vi "test Add Get and Remove Timestamp Channel.vi"(8 "error in":errorcluster, 11 "TestCase in":refnum<class "Scripting.lvclass">) -> (0 "error out":errorcluster, 3 "TestCase out":refnum<class "Scripting.lvclass">)   [LabVIEW 2020, in "Scripting.lvclass"]
uses:
  Scripting.lvclass
  <vilib>/NI VeriStand/Custom Device API/Custom Device Item Ref.ctl
  Shared/Direction.ctl
  Shared/SDI.ctl
  Scripting.lvclass/Scripting.ctl
  <vilib>/addons/_JKI Toolkits/VI Tester/TestCase.llb/TestCase.lvclass
  Scripting/AIM/AIM ARINC 429 Scripting.lvlib
  <vilib>/NI VeriStand/Custom Device API/Custom Device API.lvlib
  Shared/Transfer Speed.ctl
  C:/Program Files (x86)/National Instruments/LabVIEW 2020/vi.lib/addons/_JKI Toolkits/VI Tester/TestCase.llb/TestCase.lvclass
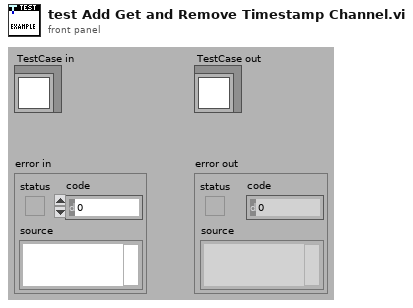
[diagram p1: front panel]
types:
  T1 = typedef "Transfer Speed.ctl" = enum16{"LO (12.5 kb/s)", "HI (100 kb/s)"}
  T2 = cluster{"SDI":bool, "SSM":bool, "Parity":bool, "Timestamp":bool}
  T3 = typedef "Direction.ctl" = enum16{"Rx", "Tx"}
  T4 = typedef "Custom Device API.lvlib/Custom Device Item Ref.ctl" = u64
  T5 = typedef "SDI.ctl" = i32
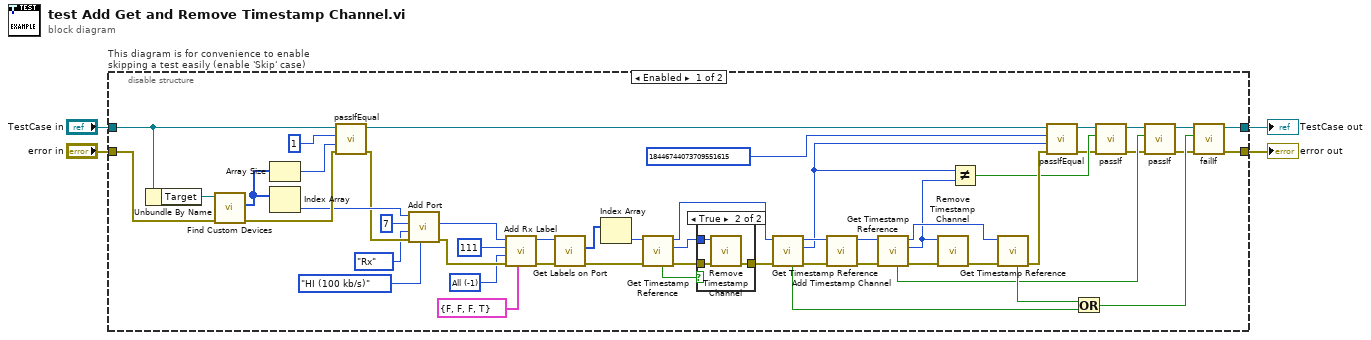
[diagram p0: block diagram]
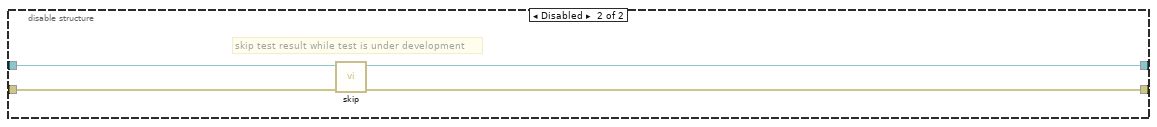
[diagram p3: hidden frame]
diagram:
  n1 = disable-structure "This diagram is for convenience to enable skipping a test easily (enable 'Skip' case)" shown="Enabled" {
    disable-tunnel: "TestCase in" -> [w55 w64]
    disable-tunnel: [w24 w62] -> w1
    disable-tunnel: [w25 w63] -> w3
    disable-tunnel: "error in" -> [w54 w61]
    frame Enabled {
      w6 = T5 -1 items=["All"=-1, "0 (b00)"=0, "1 (b01)"=1, "2 (b10)"=2, "3 (b11)"=3] ("SDI value")
      n2 = Unbundle By Name(w55) -> ("Target"=w56:refnum<k24>)
      n3 = call "Find Custom Devices.vi"("error in"=w54, "target in"=w56) -> ("error out"=w48:errorcluster, "AIM ARINC 429 custom devices"=w50:u64[])  [unwired: 7 in, 1 out]
      n4 = Array Size(array=w50) -> (size(s)=w52:i32)
      n5 = Index Array(array=w50) -> (element=w16:u64)  [unwired: 1 in]
      n6 = call-dynamic "passIfEqual.vi"("error in (no error)"=w48, "y"=w52, "x"=1 ("size(s)"), "TestCase in"=w55) -> ("error out"=w14:errorcluster, "TestCase out"=w49:refnum<class "Scripting.lvclass">)  [unwired: 6 in]
      n7 = call "Add Port.vi"("speed"=Transfer_Speed."HI (100 kb/s)", "error in"=w14, "direction"=Direction."Rx", "port number"=u16 7, "AIM ARINC 429 custom device in"=w16) -> ("error out"=w10:errorcluster, "port"=w12:T4)  [unwired: 4 in, 1 out]
      n8 = call "Add Rx Label.vi"("create channels"=T2 {"SDI"=FALSE, "SSM"=FALSE, "Parity"=FALSE, "Timestamp"=TRUE}, "error in"=w10, "SDI value"=w6, "label value"=u32 111, "port in"=w12) -> ("error out"=w9:errorcluster, "port out"=w11:T4)  [unwired: 4 in, 1 out]
      n9 = call "Get Labels on Port.vi"("error in"=w9, "port in"=w11) -> ("error out"=w31:errorcluster, "labels"=w51:T4[])  [unwired: 6 in, 2 out]
      n10 = Index Array(array=w51) -> (element=w32:T4)  [unwired: 1 in]
      n11 = call "Get Timestamp Reference.vi"("error in"=w31, "label ref in"=w32) -> ("error out"=w30:errorcluster, "timestamp channel reference"=w33:T4, "label ref out"=w29:T4, "timestamp channel found?"=w17:bool)  [unwired: 6 in]
      n12 = case shown="True" w17 {
        tunnel: w33 -> [_ w60]
        tunnel: w30 -> [w57 w59]
        tunnel: [w57 w58] -> w18
        frame False {
        }
        frame True {
          n13 = call "Remove Timestamp Channel.vi"("error in"=w59, "timestamp channel ref"=w60) -> ("error out"=w58:errorcluster)  [unwired: 9 in]
        }
      }
      n14 = call "Get Timestamp Reference.vi"("error in"=w18, "label ref in"=w29) -> ("error out"=w46:errorcluster, "timestamp channel reference"=w37:T4, "label ref out"=w47:T4, "timestamp channel found?"=w27:bool)  [unwired: 6 in]
      n15 = call "Add Timestamp Channel.vi"("error in"=w46, "label ref"=w47) -> ("error out"=w44:errorcluster, "label ref out"=w45:T4)  [unwired: 8 in]
      n16 = call "Get Timestamp Reference.vi"("error in"=w44, "label ref in"=w45) -> ("error out"=w42:errorcluster, "timestamp channel reference"=w38:T4, "label ref out"=w43:T4, "timestamp channel found?"=w23:bool)  [unwired: 6 in]
      n17 = call "Remove Timestamp Channel.vi"("error in"=w42, "timestamp channel ref"=w38) -> ("error out"=w41:errorcluster)  [unwired: 9 in]
      n18 = Not Equal?(x=w37, y=w38) -> (x != y?=w36:bool)
      n19 = call "Get Timestamp Reference.vi"("error in"=w41, "label ref in"=w43) -> ("error out"=w39:errorcluster, "timestamp channel found?"=w28:bool)  [unwired: 6 in, 2 out]
      n20 = call-dynamic "passIfEqual.vi"("error in (no error)"=w39, "y"=w37, "x"=T4 18446744073709551615 ("timestamp channel reference"), "TestCase in"=w49) -> ("error out"=w34:errorcluster, "TestCase out"=w35:refnum<class "Scripting.lvclass">)  [unwired: 6 in]
      n21 = Or(x=w28, y=w27) -> (x .or. y?=w26:bool)
      n22 = call-dynamic "passIf.vi"("error in (no error)"=w34, "pass"=w36, "TestCase in"=w35) -> ("error out"=w21:errorcluster, "TestCase out"=w22:refnum<class "Scripting.lvclass">)  [unwired: 7 in]
      n23 = call-dynamic "passIf.vi"("error in (no error)"=w21, "pass"=w23, "TestCase in"=w22) -> ("error out"=w19:errorcluster, "TestCase out"=w20:refnum<class "Scripting.lvclass">)  [unwired: 7 in]
      n24 = call-dynamic "failIf.vi"("error in (no error)"=w19, "fail"=w26, "TestCase in"=w20) -> ("error out"=w25:errorcluster, "TestCase out"=w24:refnum<class "Scripting.lvclass">)  [unwired: 7 in]
    }
    frame Disabled {
      # "skip test result while test is under development"
      n25 = call <vilib>:"skip.vi"("error in (no error)"=w61, "TestCase in"=w64) -> ("error out"=w63:errorcluster, "TestCase out"=w62:refnum<class "Scripting.lvclass">)  [unwired: 8 in]
    }
  }
  "error out" <- w3
  "TestCase out" <- w1
